vi "Check OS Version.vi"(8 "Error In":errorcluster, 10 "Warnings in":T5[](array[typedef]), 11 "Install LV Data":T1={"SSH Session"=refnum, "Status Log"="", "Detailed Log"="", "Credentials"={"Hostname or IP"="192.168.7.2", "Username"="root", "Password"=""}, "Target Info"={"OS Version"="", "CPU"="", "Systemd Version"="", "Internet Access"=FALSE, "Device Type"="", "LV Installed Ver"="", "LV Available Ver"="", "LV Upgrade Available"=FALSE, "Hostname"="", "NIC Info"=[]}, "Reboot Required?"=FALSE}) -> (0 "Error Out":errorcluster, 2 "Warnings":T5[](array[typedef]), 3 "Install LV Data":T1={"SSH Session"=refnum, "Status Log"="", "Detailed Log"="", "Credentials"={"Hostname or IP"="192.168.7.2", "Username"="root", "Password"=""}, "Target Info"={"OS Version"="", "CPU"="", "Systemd Version"="", "Internet Access"=FALSE, "Device Type"="", "LV Installed Ver"="", "LV Available Ver"="", "LV Upgrade Available"=FALSE, "Hostname"="", "NIC Info"=[]}, "Reboot Required?"=FALSE})   [LabVIEW 2014, in "LMH-LINX.lvlib"]
uses:
  <vilib>/MakerHub/LINX/LMH-LINX.lvlib
  <vilib>/MakerHub/LINX/Private/Utilties/Target Management/Install LV Data.ctl
  C:/Program Files (x86)/National Instruments/LabVIEW 2014/vi.lib/MakerHub/LINX/Resources/Renci.SshNet.dll
  Resources/Renci.SshNet.dll
  <vilib>/MakerHub/LINX/Private/Utilties/Target Management/Target Info.ctl
  <vilib>/MakerHub/LINX/Private/Utilties/Target Management/NIC Info.ctl
  <vilib>/MakerHub/LINX/Private/Utilties/Target Management/NIC Mode.ctl
  <vilib>/MakerHub/LINX/Private/Utilties/Target Management/Target Compatibility Warnings.ctl
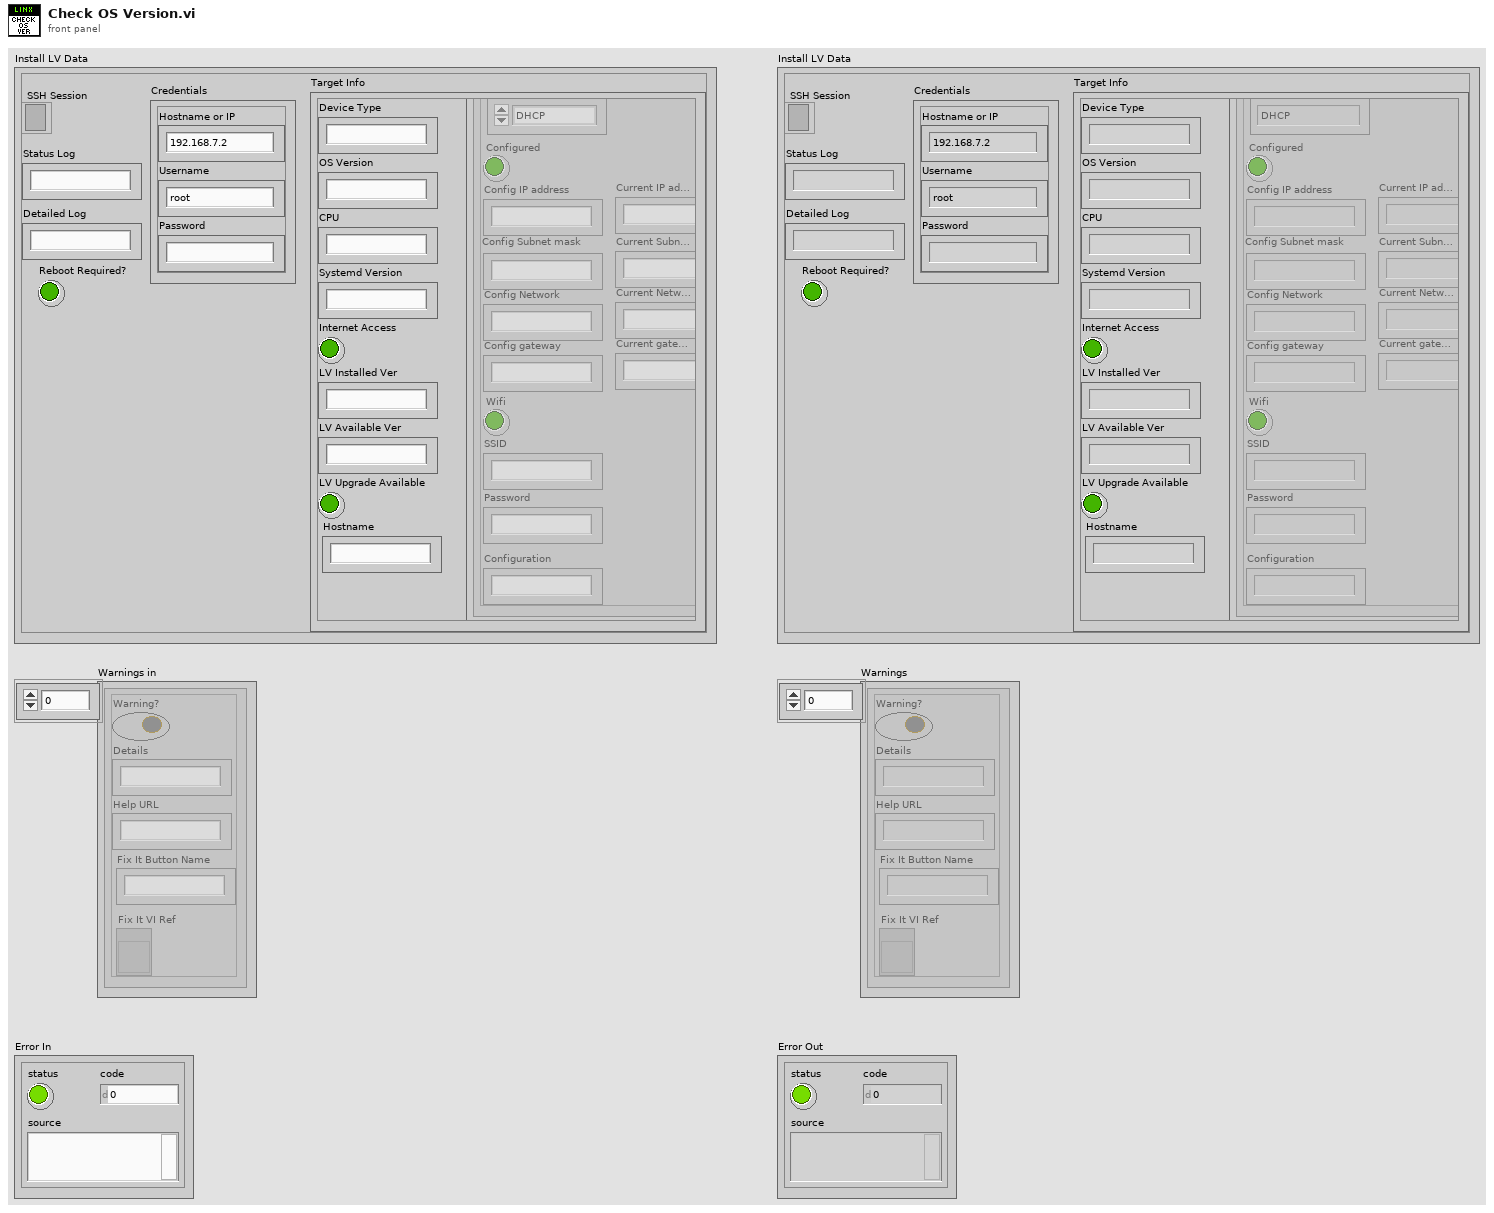
[diagram p1: front panel]
types:
  T1 = typedef "LMH-LINX.lvlib/Install LV Data.ctl" = cluster{"SSH Session":refnum<k24>, "Status Log":string, "Detailed Log":string, "Credentials":cluster{"Hostname or IP":string, "Username":string, "Password":string}, "Target Info":T2, "Reboot Required?":bool}
  T2 = typedef "LMH-LINX.lvlib/Target Info.ctl" = cluster{"OS Version":string, "CPU":string, "Systemd Version":string, "Internet Access":bool, "Device Type":string, "LV Installed Ver":string, "LV Available Ver":string, "LV Upgrade Available":bool, "Hostname":string, "NIC Info":T3[]}
  T3 = typedef "LMH-LINX.lvlib/NIC Info.ctl" = cluster{"Name":string, "NIC Mode":T4, "Configured":bool, "Config IP address":string, "Config Subnet mask":string, "Config Network":string, "Config gateway":string, "Wifi":bool, "SSID":string, "Password":string, "Configuration":string, "Current IP address":string, "Current Subnet mask":string, "Current gateway":string, "Current Network":string}
  T4 = typedef "LMH-LINX.lvlib/NIC Mode.ctl" = enum16{"DHCP", "Static", "Loopback"}
  T5 = typedef "LMH-LINX.lvlib/Target Compatibility Warnings.ctl" = cluster{"Warning?":bool, "Details":string, "Help URL":string, "Fix It Button Name":string, "Fix It VI Ref":refnum<vi>}
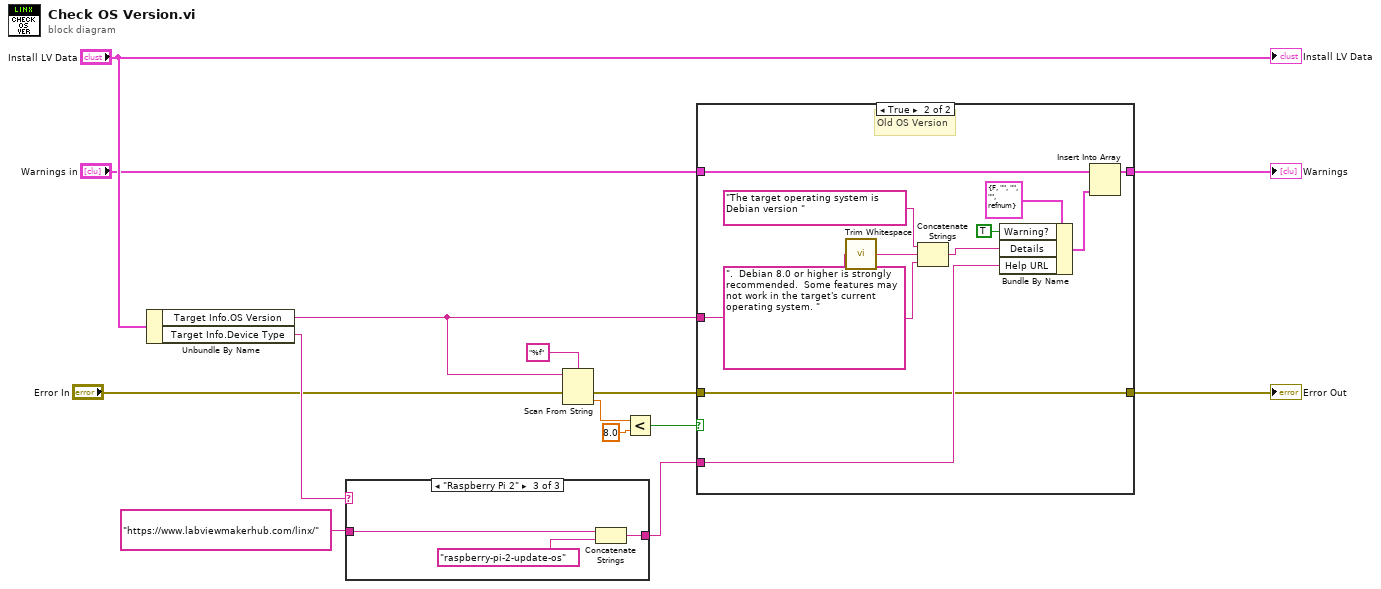
[diagram p0: block diagram]
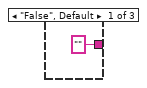
[diagram p2: hidden frame]
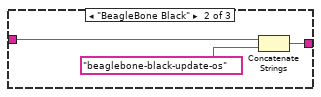
[diagram p3: hidden frame]
diagram:
  n1 = Unbundle By Name("Install LV Data") -> ("Target Info.OS Version"=w7:string, "Target Info.Device Type"=w14:string)
  n2 = case shown="\"Raspberry Pi 2\"" w14 {
    tunnel: "https://www.labviewmakerhub.com/linx/" -> [_ w18 w21]
    tunnel: ["" w16 w19] -> w9
    frame "False", Default {
    }
    frame "BeagleBone Black" {
      n3 = Concatenate Strings(w18, "beaglebone-black-update-os" ("string")) -> (w16:string)
    }
    frame "Raspberry Pi 2" {
      n4 = Concatenate Strings(w21, "raspberry-pi-2-update-os" ("string")) -> (w19:string)
    }
  }
  n5 = Scan From String(format string="%f", input string=w7, error in="Error In") -> (error out=w12:errorcluster, output 1=w4:dbl)  [unwired: 2 in, 2 out]
  n6 = Less?(x=w4, y=8.0) -> (x < y?=w2:bool)
  n7 = case shown="True" w2 {
    tunnel: w7 -> [_ w27]
    tunnel: "Warnings in" -> [w23 w33]
    tunnel: [w23 w28] -> w8
    tunnel: w9 -> [_ w25]
    tunnel: [w22 w24] -> w11
    tunnel: w12 -> [w22 w24]
    frame False {
      # "OS Version 8.x Or Newer"
    }
    frame True {
      # "Old OS Version"
      n8 = call <vilib>:"Trim Whitespace.vi"("string"=w27) -> ("trimmed string"=w26:string)  [unwired: 1 in]
      n9 = Concatenate Strings("The target operating system is Debian version ", w26, ".  Debian 8.0 or higher is strongly recommended.  Some features may not work in the target's current operating system. ") -> (w29:string)
      n10 = Bundle By Name(cluster=T5 {"Warning?"=FALSE, "Details"="", "Help URL"="", "Fix It Button Name"="", "Fix It VI Ref"=refnum} ("Target Compatibility Warnings"), "Warning?"=TRUE ("Can Continue?"), "Details"=w29, "Help URL"=w25) -> (w30:T5)
      n11 = Insert Into Array(array=w33, new element=w30) -> (w28:T5[])  [unwired: 1 in]
    }
  }
  "Error Out" <- w11
  "Warnings" <- w8
  "Install LV Data" <- "Install LV Data"
